vi "System_Update_Check.vi"(8 "error in (no error)":errorcluster, 11 "Arguments":string) -> (0 "error out":errorcluster, 2 "String":string, 3 "States Out":string)   [LabVIEW 2024]
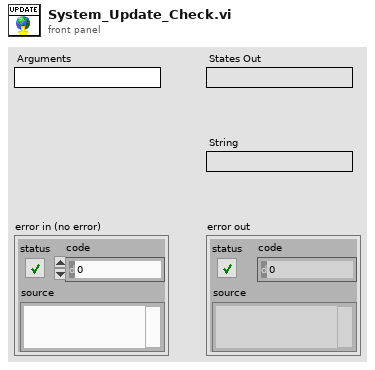
[diagram p1: front panel]
types:
  T1 = enum32{"invalid app kind", "Development System", "Run Time System", "Student Edition", "Embedded LabVIEW", "Evaluation", "Custom"}
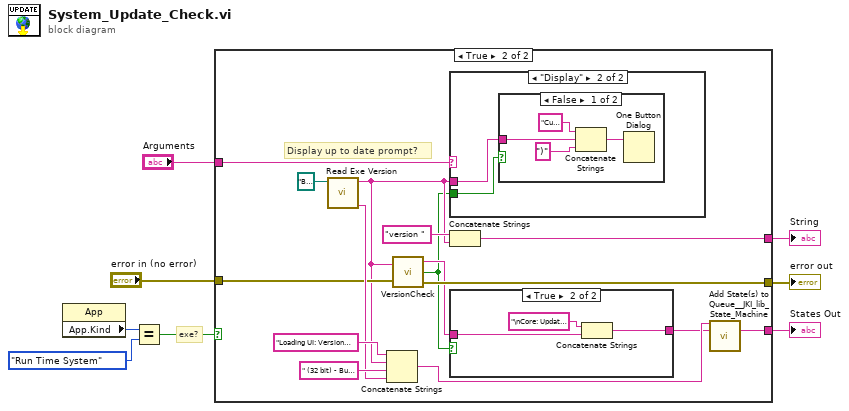
[diagram p0: block diagram]
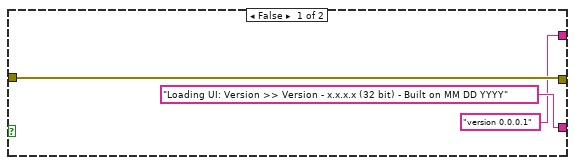
[diagram p2: hidden frame]
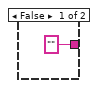
[diagram p5: hidden frame]
diagram:
  # "exe?"
  n1 = property class="App"() -> ("App.Kind"=w4:T1)  [unwired: 2 in, 2 out]
  n2 = Equal?(x=w4, y=T1."Run Time System" ("Application:Kind")) -> (x = y?=w5:bool)
  n3 = case shown="True" w5 {
    tunnel: "error in (no error)" -> [w11 w22]
    tunnel: [w11 w21] -> w2
    tunnel: ["Loading UI: Version >> Version - x.x.x.x (32 bit) - Built on MM DD YYYY" w18] -> w6
    tunnel: "Arguments" -> [_ w17]
    tunnel: ["version 0.0.0.1" w12] -> w8
    frame False {
    }
    frame True {
      # "Display up to date prompt?"
      n4 = call "Read Exe Version.vi"("Application name"=path "BioSIM.exe") -> ("Build Date"=w23:string, "FileVersion"=w15:string)  [unwired: 7 in, 2 out]
      n5 = Concatenate Strings("Loading UI: Version >> Version - " ("string"), w15, " (32 bit) - Built on " ("string"), w23) -> (w20:string)
      n6 = call "VersionCheck.vi"("Version"=w15, "error in (no error)"=w22) -> ("Latest Version"=w16:string, "outdated?"=w14:bool, "error out"=w21:errorcluster)
      n7 = case shown="\"Display\"" w17 {
        tunnel: w15 -> [_ w28]
        tunnel: w14 -> [_ w27]
        frame "False", Default {
        }
        frame "Display" {
          n8 = case shown="False" w27 {
            tunnel: w28 -> [w31 _]
            frame False {
              n9 = Concatenate Strings("Current version is the latest (" ("message"), w31, ")" ("string")) -> (w29:string)
              n10 = One Button Dialog(message=w29) -> ()  [unwired: 1 in, 1 out]
            }
            frame True {
            }
          }
        }
      }
      n11 = Concatenate Strings("version " ("string"), w15) -> (w12:string)
      n12 = case shown="True" w14 {
        tunnel: ["" w34] -> w19
        tunnel: w16 -> [_ w35]
        frame False {
        }
        frame True {
          n13 = Concatenate Strings("\nCore: Update >> " ("string"), w35) -> (w34:string)
        }
      }
      n14 = call <vilib>:"Add State(s) to Queue__JKI_lib_State_Machine.vi"("State(s) in Front (\"\")"=w20, "State(s) in (\"\")"=w19) -> ("States Out"=w18:string)  [unwired: 13 in]
    }
  }
  "String" <- w8
  "States Out" <- w6
  "error out" <- w2
